vi "CMD_JOYSTICK.vi"(6 "Gantry in":refnum<class "Gantry.lvclass">, 8 "error in (no error)":errorcluster, 10 "Arguments":string[](array[string]), 11 "gScript Interpreter in":refnum<class "gScript Interpreter.lvclass">) -> (0 "error out":errorcluster, 3 "gScript Interpreter out":refnum<class "gScript Interpreter.lvclass">, 4 "Gantry out":refnum<class "Gantry.lvclass">)   [LabVIEW 2017, in "gScript Interpreter.lvclass"]
uses:
  gScript Interpreter.lvclass
  Shared Components/Gantry Class/Gantry.lvclass
panel:
  in  "Finished?":bool=TRUE
  out "Preview":T1(plugin-control)
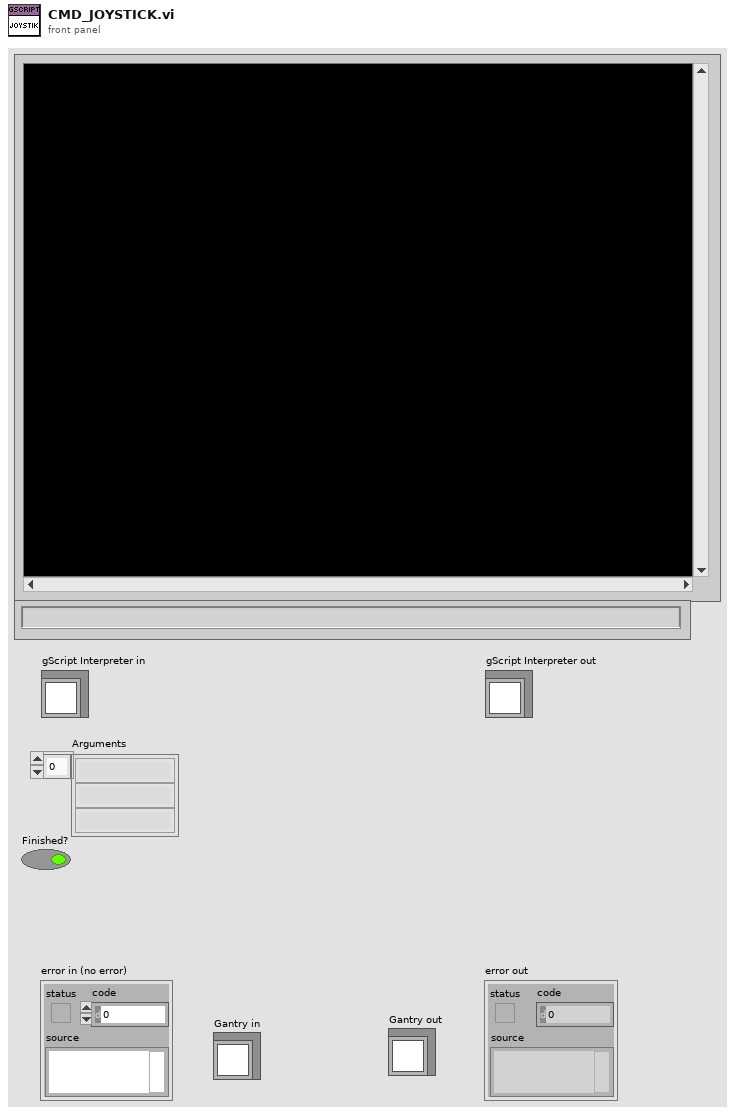
[diagram p1: front panel]
types:
  T1 = typedef "IMAQ Image.ctl" = refnum<image>
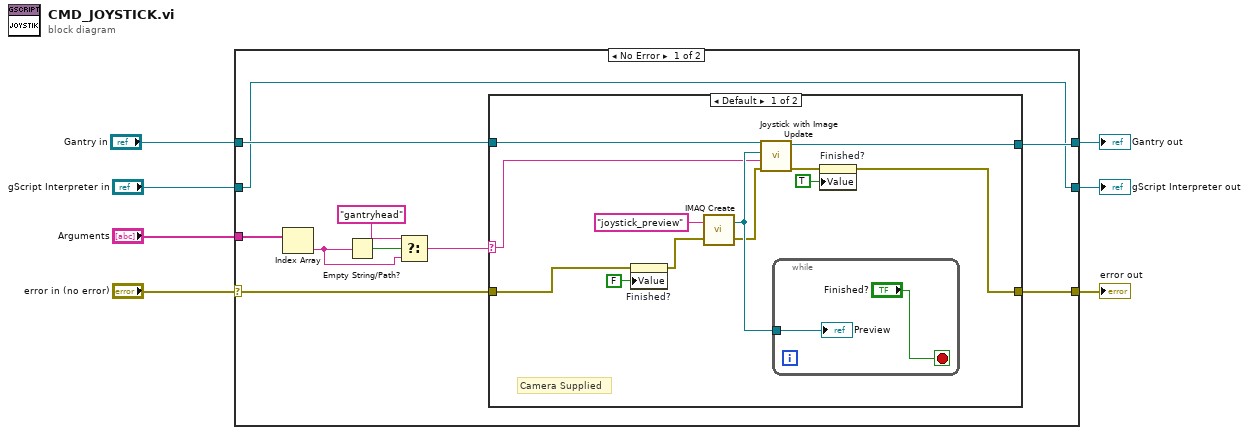
[diagram p0: block diagram]
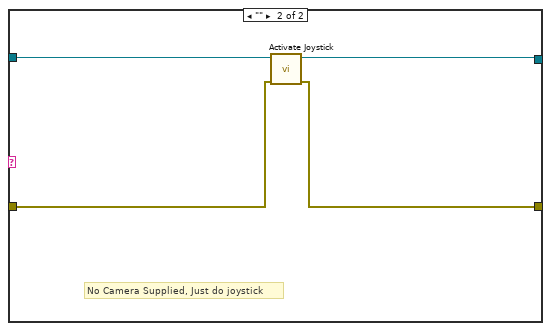
[diagram p2: hidden frame]
diagram:
  n1 = case shown="No Error" "error in (no error)" {
    selector: "error in (no error)" -> [w12 w38]
    tunnel: [w14 w38] -> w6
    tunnel: [w13 w37] -> w4
    tunnel: "gScript Interpreter in" -> [w13 w37]
    tunnel: "Arguments" -> [w17 _]
    tunnel: "Gantry in" -> [w16 w36]
    tunnel: [w15 w36] -> w1
    frame No Error {
      n2 = Index Array(array=w17) -> (element=w9:string)  [unwired: 1 in]
      n3 = Empty String/Path?(string/path=w9) -> (empty?=w11:bool)
      n4 = Select(t="gantryhead", s=w11, f=w9) -> (s? t:f=w8:string)
      n5 = case shown="Default" w8 {
        selector: w8 -> [w19 _]
        tunnel: w16 -> [w29 w35]
        tunnel: [w26 w34] -> w15
        tunnel: [w20 w33] -> w14
        tunnel: w12 -> [w18 w32]
        frame Default {
          # "Camera Supplied"
          n6 = property on="Finished?" class="Bool (strict)"(error in=w18, "Value"=FALSE ("Finished?")) -> (error out=w25:errorcluster)  [unwired: 1 in, 1 out]
          n7 = call "IMAQ Create"("Image Name"="joystick_preview", "error in (no error)"=w25) -> ("New Image"=w27:T1, "error out"=w21:errorcluster)  [unwired: 3 in]
          n8 = call-dynamic "Joystick with Image Update.vi"("error in (no error)"=w21, "Camera Name"=w19, "Image In"=w27, "Gantry Class in"=w29) -> ("error out"=w24:errorcluster, "Gantry Class out"=w26:refnum<class "Gantry.lvclass">)  [unwired: 5 in, 1 out]
          n9 = while {
            tunnel: w27 -> [w31]
            stop <- "Finished?" stop-if-true
            "Preview" <- w31
          }
          n10 = property on="Finished?" class="Bool (strict)"(error in=w24, "Value"=TRUE ("Finished?")) -> (error out=w20:errorcluster)  [unwired: 1 in, 1 out]
        }
        frame "" {
          # "No Camera Supplied, Just do joystick"
          n11 = call-dynamic "Activate Joystick.vi"("error in (no error)"=w32, "Gantry Class in"=w35) -> ("error out"=w33:errorcluster, "Gantry Class out"=w34:refnum<class "Gantry.lvclass">)  [unwired: 8 in]
        }
      }
    }
    frame Error {
    }
  }
  "error out" <- w6
  "gScript Interpreter out" <- w4
  "Gantry out" <- w1
